vi "Process MIDI.vi"(8 "error in (no error)":errorcluster) -> (0 "error out":errorcluster)   [LabVIEW 2014]
uses:
  MIDI driver/MID Command.ctl
panel:
  out "Numeric":i32
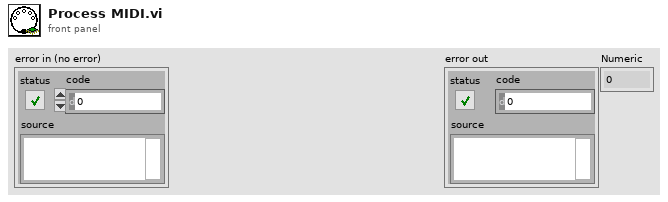
[diagram p1: front panel]
types:
  T1 = typedef "MID Command.ctl" = cluster{"Device":enum16{"Keys", "Controls", "Pads"}, "Parameter 1":u8, "Parameter 2":u8}
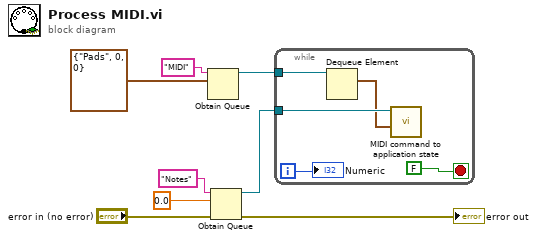
[diagram p0: block diagram]
diagram:
  n1 = Obtain Queue(name (unnamed)="MIDI", element data type=T1 {"Device"=enum."Pads", "Parameter 1"=0, "Parameter 2"=0} ("MIDI Command")) -> (queue out=w3:refnum<queue>)  [unwired: 3 in, 2 out]
  n2 = Obtain Queue(name (unnamed)="Notes", element data type=0.0, error in (no error)="error in (no error)") -> (queue out=w4:refnum<queue>, error out=→"error out":errorcluster)  [unwired: 2 in, 1 out]
  n3 = while {
    tunnel: w4 -> [w13]
    tunnel: w3 -> [w12]
    i -> [w9]
    stop <- FALSE stop-if-true
    n4 = Dequeue Element(queue=w12) -> (element=w11:T1)  [unwired: 2 in, 3 out]
    n5 = call "MIDI command to application state.vi"("MIDI Command"=w11, "Note Queue"=w13) -> ()  [unwired: 10 in]
    "Numeric" <- w9
  }
